vi "DBL.vi"(4 "Value":T1) -> (1 "Constant":refnum<class "Const_I8.lvclass">)   [LabVIEW 2021, in "Const_I8.lvclass"]
uses:
  Const_I8.lvclass
  Type.ctl
  Const_I8.lvclass/Const_I8.ctl
  Properties/Write Value.vi
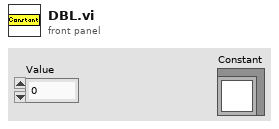
[diagram p1: front panel]
types:
  T1 = typedef "Const_I8.lvclass/Type.ctl" = dbl
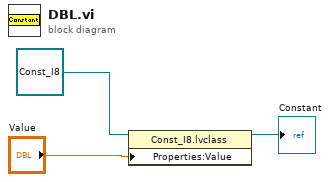
[diagram p0: block diagram]
diagram:
  n1 = property class="Const_I8.lvclass"(reference=refnum<class "Const_I8.lvclass"> refnum ("Constants.lvlib:Numeric.lvclass"), "Properties:Value"="Value") -> (reference out=→"Constant":refnum<class "Const_I8.lvclass">)  [unwired: 1 in, 1 out]
